vi "GetOperation.vi"(6 "Timeout in ms (-1)":i32, 8 "error in (no error)":errorcluster, 11 "SMP in":refnum<class "SMP.lvclass">) -> (0 "error out":errorcluster, 1 "Previous data":variant, 2 "Operation":T1, 3 "SMP out":refnum<class "SMP.lvclass">, 4 "Timed out?":bool, 5 "Pipe operation?":bool)   [LabVIEW 2013, in "SMP.lvclass"]
doc: "Returns an operation from the front of the operations queue of the SMP object.\n\n<b>Timeout: </b>A timeout for the dequeue operation. Default is -1 (never time out).\n\n<b>Pipe operation: </b>TRUE if the returned operation is part of a pipe. FALSE otherwise.\n\n<b>Operation: </b>The returned operation. This can be either an individual operation or an operation which is part of a pipe.\n\n<b>Previous data: </b>Data which was produced by the previous operation in the queue. This must be explicitly set using the function SetPreviousData, after the previous operation has completed.\n\n<b>Timed out: </b>TRUE if the dequeue operation timed out. FALSE otherwise."
uses:
  SMP.lvclass
  Data types/operation.ctl
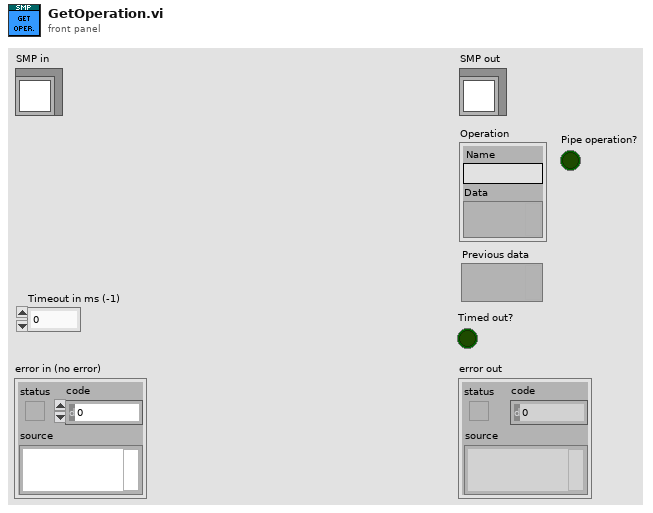
[diagram p1: front panel]
types:
  T1 = typedef "SMP.lvclass/operation.ctl" = cluster{"Name":string, "Data":variant}
  T2 = typedef "Pipe and Filter.lvclass/classData.ctl" = cluster{"Q ref":refnum<queue>, "Previous data":variant, "Current pipe":T3[]}
  T3 = typedef "Pipe and Filter.lvclass/operation.ctl" = cluster{"Name":string, "Data":variant}
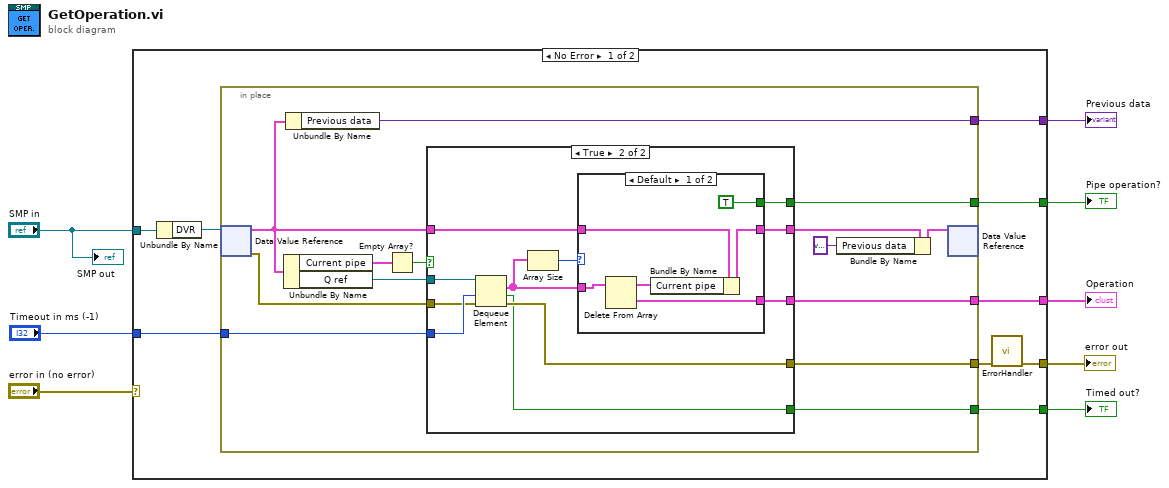
[diagram p0: block diagram]
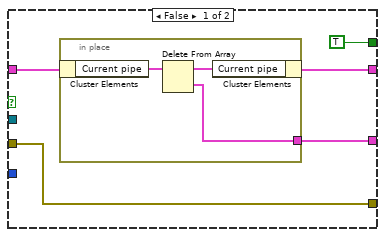
[diagram p2: hidden frame]
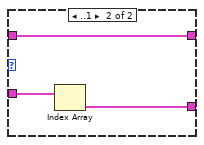
[diagram p3: hidden frame]
diagram:
  n1 = case shown="No Error" "error in (no error)" {
    selector: "error in (no error)" -> [_ w60]
    tunnel: [w14 w60] -> w7
    tunnel: "SMP in" -> [w16 _]
    tunnel: "Timeout in ms (-1)" -> [w13 _]
    tunnel: [w12 _] -> w4
    tunnel: [w11 _] -> w3
    tunnel: [w10 _] -> w2
    tunnel: [w9 _] -> w1
    frame No Error {
      n2 = Unbundle By Name(w16) -> ("DVR"=w17:refnum<data-value>)
      n3 = in-place {
        in-place-border: [w29] -> w15
        in-place-border: w13 -> [w31]
        in-place-border: [w25] -> w12
        in-place-border: [w22] -> w11
        in-place-border: [w19] -> w10
        in-place-border: [w18] -> w9
        n4 = in-place-dvr #1(w17) -> (w24:T2, w30:errorcluster)
        n5 = Unbundle By Name(w24) -> ("Current pipe"=w26:T3[], "Q ref"=w28:refnum<queue>)
        n6 = Unbundle By Name(w24) -> ("Previous data"=w25:variant)
        n7 = Empty Array?(array=w26) -> (empty?=w27:bool)
        n8 = case shown="True" w27 {
          tunnel: w31 -> [_ w50]
          tunnel: w30 -> [w33 w49]
          tunnel: [w33 w48] -> w29
          tunnel: w28 -> [_ w47]
          tunnel: w24 -> [w35 w43]
          tunnel: [w34 w42] -> w23
          tunnel: [w36 w44] -> w22
          tunnel: [TRUE w40] -> w19
          tunnel: [_ w41] -> w18
          frame False {
            n9 = in-place {
              in-place-border: [w39] -> w36
              n10 = in-place-cluster #2(w35) -> ("Current pipe"=w38:T3[])
              n11 = Delete From Array(array=w38) -> (deleted portion=w39:T3, array with subset deleted=w37:T3[])  [unwired: 2 in]
              n12 = in-place-cluster #2("Current pipe"=w37) -> (w34:T2)
            }
          }
          frame True {
            n13 = Dequeue Element(queue=w47, timeout in ms (-1)=w50, error in (no error)=w49) -> (element=w45:T3[], timed out?=w41:bool, error out=w48:errorcluster)  [unwired: 1 out]
            n14 = Array Size(array=w45) -> (size(s)=w46:i32)
            n15 = case shown="Default" w46 {
              tunnel: w45 -> [w52 w59]
              tunnel: [w55 w58] -> w44
              tunnel: w43 -> [w53 w57]
              tunnel: [w56 w57] -> w42
              tunnel: [TRUE _] -> w40
              frame Default {
                n16 = Delete From Array(array=w52) -> (deleted portion=w55:T3, array with subset deleted=w54:T3[])  [unwired: 2 in]
                n17 = Bundle By Name(cluster=w53, "Current pipe"=w54) -> (w56:T2)
              }
              frame ..1 {
                n18 = Index Array(array=w59) -> (element=w58:T3)  [unwired: 1 in]
              }
            }
          }
        }
        n19 = Bundle By Name(cluster=w23, "Previous data"=variant) -> (w21:T2)
        n20 = in-place-dvr #1(w21) -> ()  [unwired: 2 out]
      }
      n21 = call "ErrorHandler.vi"("error in (no error)"=w15) -> ("error out"=w14:errorcluster)  [unwired: 9 in, 1 out]
    }
    frame Error {
    }
  }
  "error out" <- w7
  "Previous data" <- w4
  "Operation" <- w3
  "Pipe operation?" <- w2
  "Timed out?" <- w1
  "SMP out" <- "SMP in"
